vi "Read RelatedIssues.vi"(8 "error in (no error)":errorcluster, 11 "Component in":refnum<class "Component.lvclass">) -> (0 "error out":errorcluster, 2 "RelatedIssues":dbl, 3 "Component out":refnum<class "Component.lvclass">)   [LabVIEW 2018, in "Component.lvclass"]
uses:
  Component.lvclass
  Component.lvclass/Component.ctl
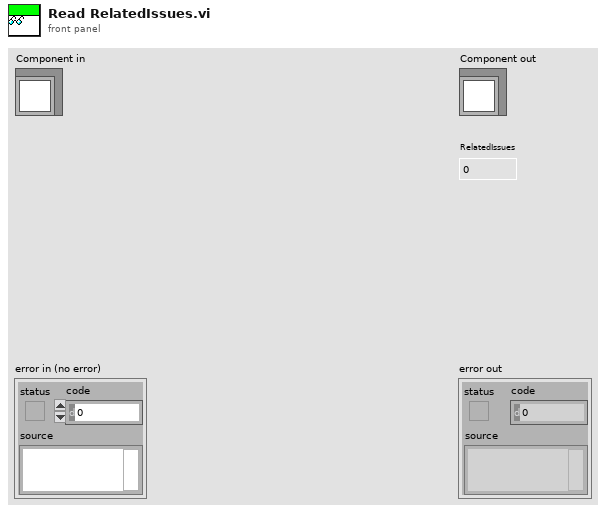
[diagram p1: front panel]
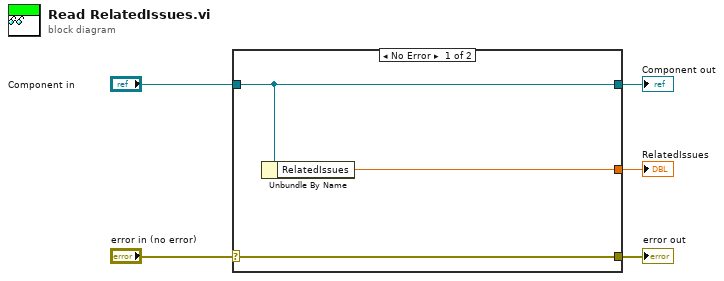
[diagram p0: block diagram]
diagram:
  n1 = case shown="No Error" "error in (no error)" {
    selector: "error in (no error)" -> [w8 w9]
    tunnel: [w8 w9] -> w4
    tunnel: [w7 w10] -> w2
    tunnel: "Component in" -> [w7 w10]
    tunnel: [w6 _] -> w1
    frame No Error {
      n2 = Unbundle By Name(w7) -> ("RelatedIssues"=w6:dbl)
    }
    frame Error {
    }
  }
  "error out" <- w4
  "Component out" <- w2
  "RelatedIssues" <- w1
